vi "SV Remove Delays (1,N) from Waveforms (N Ch) (DBL).vi"(7 "reset":bool, 8 "error in (no error)":errorcluster, 9 "path-dependent analog delays [s]":dbl[](array[numeric]) format="%.2p", 10 "shared digital delay [samples]":dbl min=0.0 format="%.1f", 11 "scaled signals":waveform(dbl)[](array[waveform])) -> (0 "error out":errorcluster, 1 "residual delays [s]":dbl[](array[numeric]) format="%.2p", 2 "aligned signals length":i32, 3 "aligned signals":waveform(dbl)[](array[waveform]))   [LabVIEW 2017]
doc: "Use this VI to align waveforms for channels with propagation delay. For each channel, signal delay is added such that all signals have the same (maximum) delay. This common delay is then removed from all signals. This VI maintains a FIFO for each channel to keep the signals aligned with subsequent calls to the VI. The output waveforms will all have the same length. This VI may output waveforms with a different length on reset=TRUE or first call than in subsequent calls."
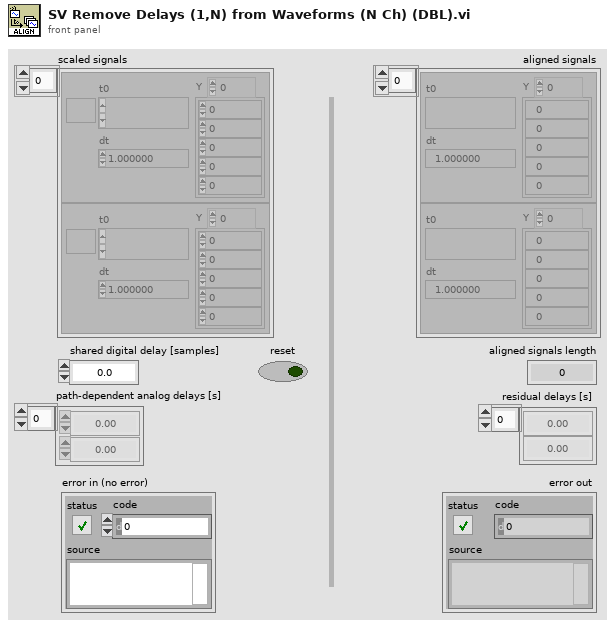
[diagram p1: front panel]
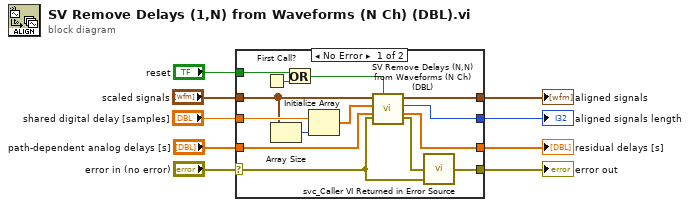
[diagram p0: block diagram]
diagram:
  n1 = case shown="No Error" "error in (no error)" {
    selector: "error in (no error)" -> [w10 w24]
    tunnel: "scaled signals" -> [w21 _]
    tunnel: "shared digital delay [samples]" -> [w22 _]
    tunnel: "path-dependent analog delays [s]" -> [w18 _]
    tunnel: [w14 _] -> w5
    tunnel: [w12 _] -> w4
    tunnel: "reset" -> [w16 _]
    tunnel: [w23 w24] -> w2
    tunnel: [w13 _] -> w1
    frame No Error {
      n2 = First Call?() -> (First Call?: T/F=w17:bool)
      n3 = Array Size(array=w21) -> (size(s)=w20:i32)
      n4 = Or(x=w16, y=w17) -> (x .or. y?=w15:bool)
      n5 = Initialize Array(w22, w20) -> (w19:dbl[])
      n6 = call <vilib>:"SV Remove Delays (N,N) from Waveforms (N Ch) (DBL).vi"("reset"=w15, "error in (no error)"=w10, "path-dependent analog delays [s]"=w18, "channel-dependent digital delays [samples]"=w19, "scaled signals"=w21) -> ("error out"=w11:errorcluster, "residual delays [s]"=w12:dbl[], "aligned signals length"=w13:i32, "aligned signals"=w14:waveform(dbl)[])  [unwired: 3 in]
      n7 = call <vilib>:"svc_Caller VI Returned in Error Source.vi"("warning input to caller"=w10, "error in (no error)"=w11) -> ("error out"=w23:errorcluster)  [unwired: 3 in]
    }
    frame Error {
    }
  }
  "aligned signals" <- w5
  "error out" <- w2
  "residual delays [s]" <- w4
  "aligned signals length" <- w1
